vi "NET_PDPStatus.vi"(8 "Read(F) Write(T)":bool, 11 "PDP_Status_In":T1) -> (3 "PDP_Status_Out":T1)   [LabVIEW 2017]
uses:
  RoboRio code/TypeDef/CLUSTER_PDP_Status.ctl
  RoboRio code/TypeDef/CLUSTER_PDP_Faults.ctl
  <vilib>/Rock Robotics/Network Tables/NT Read Boolean Array.vi
  <vilib>/Rock Robotics/Network Tables/NT Read Numeric Array.vi
  <vilib>/Rock Robotics/Network Tables/NT Write Boolean Array.vi
  <vilib>/Rock Robotics/Network Tables/NT Write Numeric Array.vi
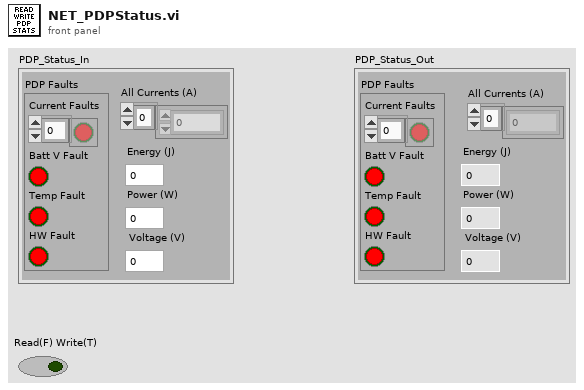
[diagram p1: front panel]
types:
  T1 = typedef "CLUSTER_PDP_Status.ctl" = cluster{"PDP Faults":T2, "All Currents (A)":dbl[], "Energy (J)":dbl, "Power (W)":dbl, "Voltage (V)":dbl}
  T2 = typedef "CLUSTER_PDP_Faults.ctl" = cluster{"Current Faults":bool[], "Batt V Fault":bool, "Temp Fault":bool, "HW Fault":bool}
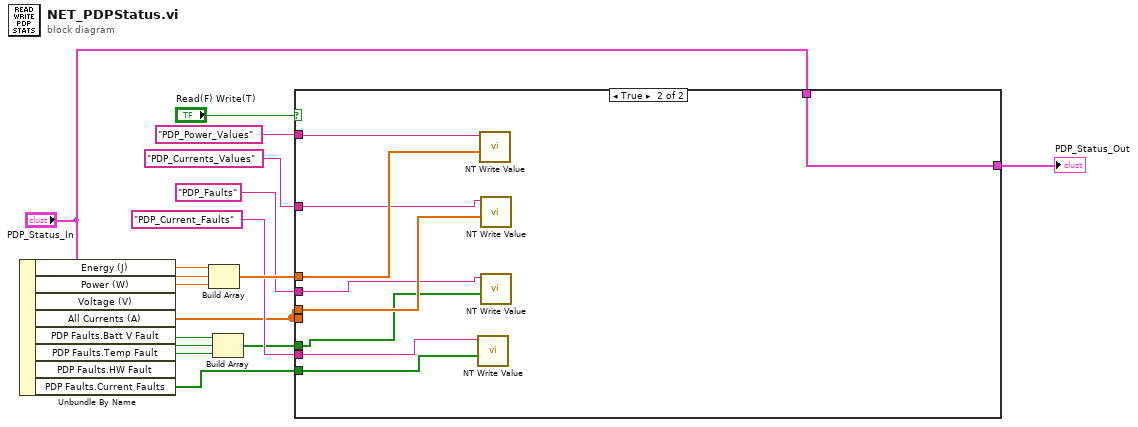
[diagram p0: block diagram]
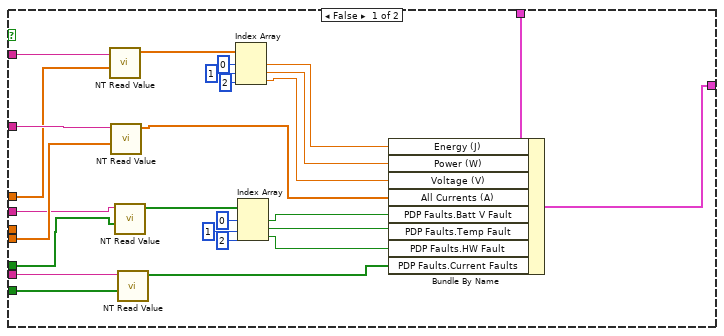
[diagram p2: hidden frame]
diagram:
  n1 = Unbundle By Name("PDP_Status_In") -> ("Energy (J)"=w14:dbl, "Power (W)"=w13:dbl, "Voltage (V)"=w12:dbl, "All Currents (A)"=w1:dbl[], "PDP Faults.Batt V Fault"=w9:bool, "PDP Faults.Temp Fault"=w8:bool, "PDP Faults.HW Fault"=w7:bool, "PDP Faults.Current Faults"=w3:bool[])
  n2 = Build Array(w14, w13, w12) -> (w10:dbl[])
  n3 = Build Array(w9, w8, w7) -> (w4:bool[])
  n4 = case shown="True" "Read(F) Write(T)" {
    tunnel: "PDP_Power_Values" ("Name") -> [w43 w48]
    tunnel: [w18 w44] -> w15
    tunnel: "PDP_Currents_Values" ("Name") -> [w42 w47]
    tunnel: w10 -> [w41 w52]
    tunnel: w1 -> [w40 _]
    tunnel: "PDP_Faults" ("Name") -> [w39 w46]
    tunnel: "PDP_Current_Faults" ("Name") -> [w38 w45]
    tunnel: w4 -> [w37 w50]
    tunnel: w3 -> [w36 w49]
    tunnel: "PDP_Status_In" -> [w26 w44]
    tunnel: w1 -> [_ w51]
    frame False {
      n5 = call-poly <vilib>:"NT Read Value.vi"("Default Value"=w41, "Name"=w43) -> ("Numeric Array"=w34:dbl[])  [unwired: 8 in, 1 out]
      n6 = call-poly <vilib>:"NT Read Value.vi"("Default Value"=w40, "Name"=w42) -> ("Numeric Array"=w23:dbl[])  [unwired: 8 in, 1 out]
      n7 = call-poly <vilib>:"NT Read Value.vi"("Default Value"=w37, "Name"=w39) -> ("Boolean Array"=w35:bool[])  [unwired: 8 in, 1 out]
      n8 = call-poly <vilib>:"NT Read Value.vi"("Default Value"=w36, "Name"=w38) -> ("Boolean Array"=w19:bool[])  [unwired: 8 in, 1 out]
      n9 = Index Array(array=w34, index #1=0 ("index"), index #2=1 ("index"), index #3=2 ("index")) -> (element #1=w27:dbl, element #2=w25:dbl, element #3=w24:dbl)
      n10 = Index Array(array=w35, index #1=0 ("index"), index #2=1 ("index"), index #3=2 ("index")) -> (element #1=w22:bool, element #2=w21:bool, element #3=w20:bool)
      n11 = Bundle By Name(cluster=w26, "Energy (J)"=w27, "Power (W)"=w25, "Voltage (V)"=w24, "All Currents (A)"=w23, "PDP Faults.Batt V Fault"=w22, "PDP Faults.Temp Fault"=w21, "PDP Faults.HW Fault"=w20, "PDP Faults.Current Faults"=w19) -> (w18:T1)
    }
    frame True {
      n12 = call-poly <vilib>:"NT Write Value.vi"("Boolean Array"=w49, "Name"=w45) -> ()  [unwired: 9 in, 1 out]
      n13 = call-poly <vilib>:"NT Write Value.vi"("Numeric Array"=w52, "Name"=w48) -> ()  [unwired: 9 in, 1 out]
      n14 = call-poly <vilib>:"NT Write Value.vi"("Numeric Array"=w51, "Name"=w47) -> ()  [unwired: 9 in, 1 out]
      n15 = call-poly <vilib>:"NT Write Value.vi"("Boolean Array"=w50, "Name"=w46) -> ()  [unwired: 9 in, 1 out]
    }
  }
  "PDP_Status_Out" <- w15
